vi "Next is Authority Slashes.vi"(1 "Constructor String Parser":T1) -> (0 "Authority Slashes":bool)   [LabVIEW 2020, in "Stream.lvlib" / "URLPattern.lvclass"]
uses:
  URLPattern.lvclass
  Token Type.ctl
  Token.ctl
  URL Pattern Init.ctl
  Parser State.ctl
  Constructor String Parser.ctl
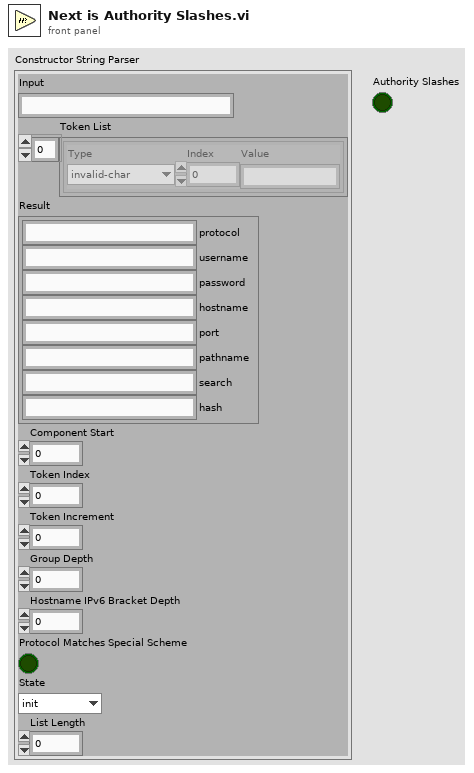
[diagram p1: front panel]
types:
  T1 = typedef "Stream.lvlib/URLPattern.lvclass/Constructor String Parser.ctl" = cluster{"Input":string, "Token List":T2[], "Result":T4, "Component Start":i32, "Token Index":i32, "Token Increment":i32, "Group Depth":i32, "Hostname IPv6 Bracket Depth":i32, "Protocol Matches Special Scheme":bool, "State":T5, "List Length":i32}
  T2 = typedef "Stream.lvlib/URLPattern.lvclass/Token.ctl" = cluster{"Type":T3, "Index":i32, "Value":string}
  T3 = typedef "Stream.lvlib/URLPattern.lvclass/Token Type.ctl" = enum16{"invalid-char", "open", "close", "regexp", "name", "char", "escaped-char", "other-modifier", "asterisk", "end"}
  T4 = typedef "Stream.lvlib/URLPattern.lvclass/URL Pattern Init.ctl" = cluster{"protocol":string, "username":string, "password":string, "hostname":string, "port":string, "pathname":string, "search":string, "hash":string}
  T5 = typedef "Stream.lvlib/URLPattern.lvclass/Parser State.ctl" = enum16{"init", "protocol", "authority", "username", "password", "hostname", "port", "pathname", "search", "hash", "done"}
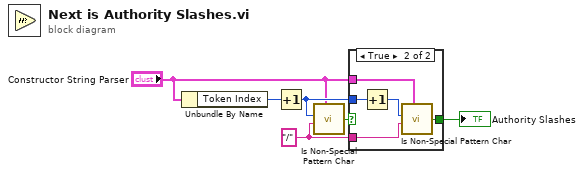
[diagram p0: block diagram]
diagram:
  w1 = "/" ("Value")
  n1 = Unbundle By Name("Constructor String Parser") -> ("Token Index"=w6:i32)
  n2 = Increment(x=w6) -> (x+1=w3:i32)
  n3 = call "Is Non-Special Pattern Char.vi"("Value"=w1, "Constructor String Parser"="Constructor String Parser", "Index"=w3) -> ("Non-Special Pattern Char?"=w5:bool)  [unwired: 7 in]
  n4 = case shown="True" w5 {
    selector: w5 -> [w7 _]
    tunnel: [w7 w8] -> w4
    tunnel: w3 -> [_ w12]
    tunnel: "Constructor String Parser" -> [_ w10]
    tunnel: w1 -> [_ w9]
    frame False {
    }
    frame True {
      n5 = Increment(x=w12) -> (x+1=w11:i32)
      n6 = call "Is Non-Special Pattern Char.vi"("Value"=w9, "Constructor String Parser"=w10, "Index"=w11) -> ("Non-Special Pattern Char?"=w8:bool)  [unwired: 7 in]
    }
  }
  "Authority Slashes" <- w4
